vi "SerialSendHLcmd.vi"(0 "ASI stage":T1, 1 "Axis configuration":u16(ring) items=["No axis", "X", "Y", "Z", "XY", "XYZ"], 5 "Command":string, 7 "data in":cluster{"X in":dbl, "Y in":dbl, "Z in":dbl} {"Z in" format="%#.4f"; "Y in" format="%#.4f"; "X in" format="%#.4f"}, 11 "error in (no error)":errorcluster, 12 "Command type":enum16{"Query", "Where", "Imperative", "DU Y"}(ring)) -> (4 "Raw receive buffer":string, 6 "data out":cluster{"X out":dbl, "Y out":dbl, "Z out":dbl} {"Z out" format="%#.4f"; "Y out" format="%#.4f"; "X out" format="%#.4f"}, 15 "error out":errorcluster)   [LabVIEW 2010]
uses:
  stage properties.ctl
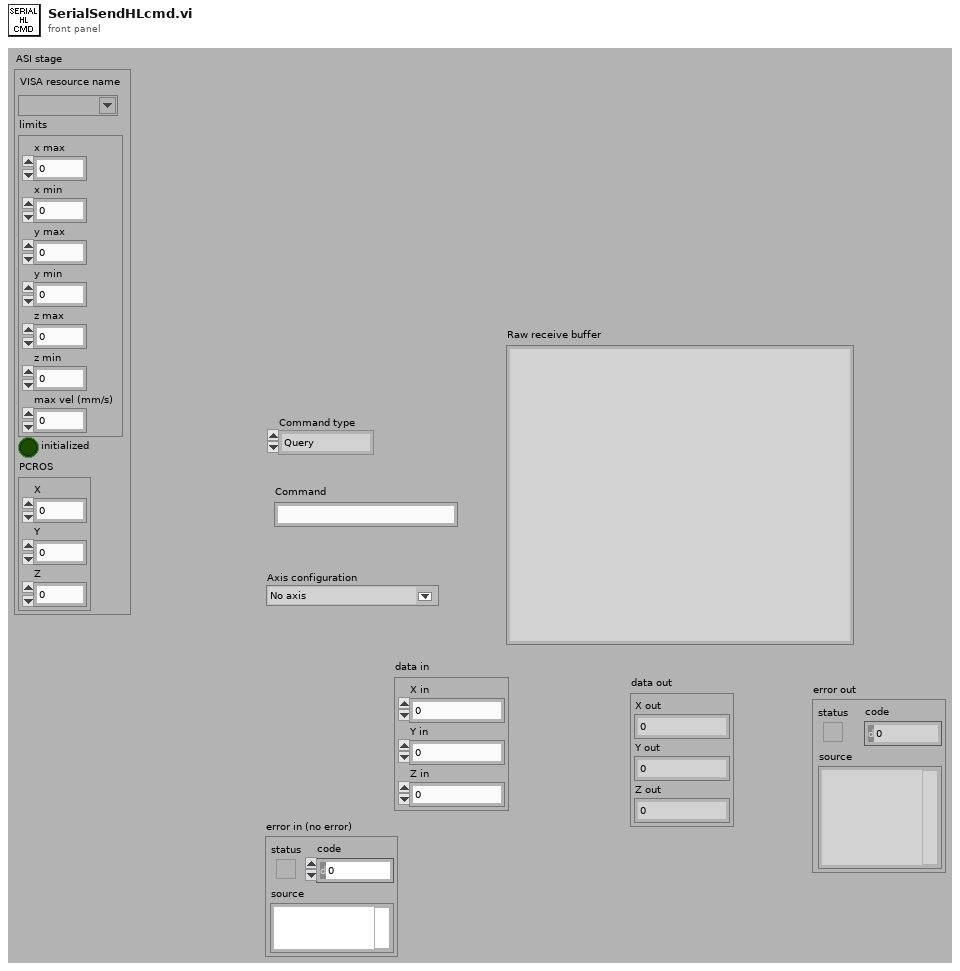
[diagram p1: front panel]
types:
  T1 = typedef "stage properties.ctl" = cluster{"VISA resource name":refnum<visa-resource-name>, "limits":cluster{"x max":dbl, "x min":dbl, "y max":dbl, "y min":dbl, "z max":dbl, "z min":dbl, "max vel (mm/s)":dbl}, "initialized":bool, "PCROS":cluster{"X":dbl, "Y":dbl, "Z":dbl}}
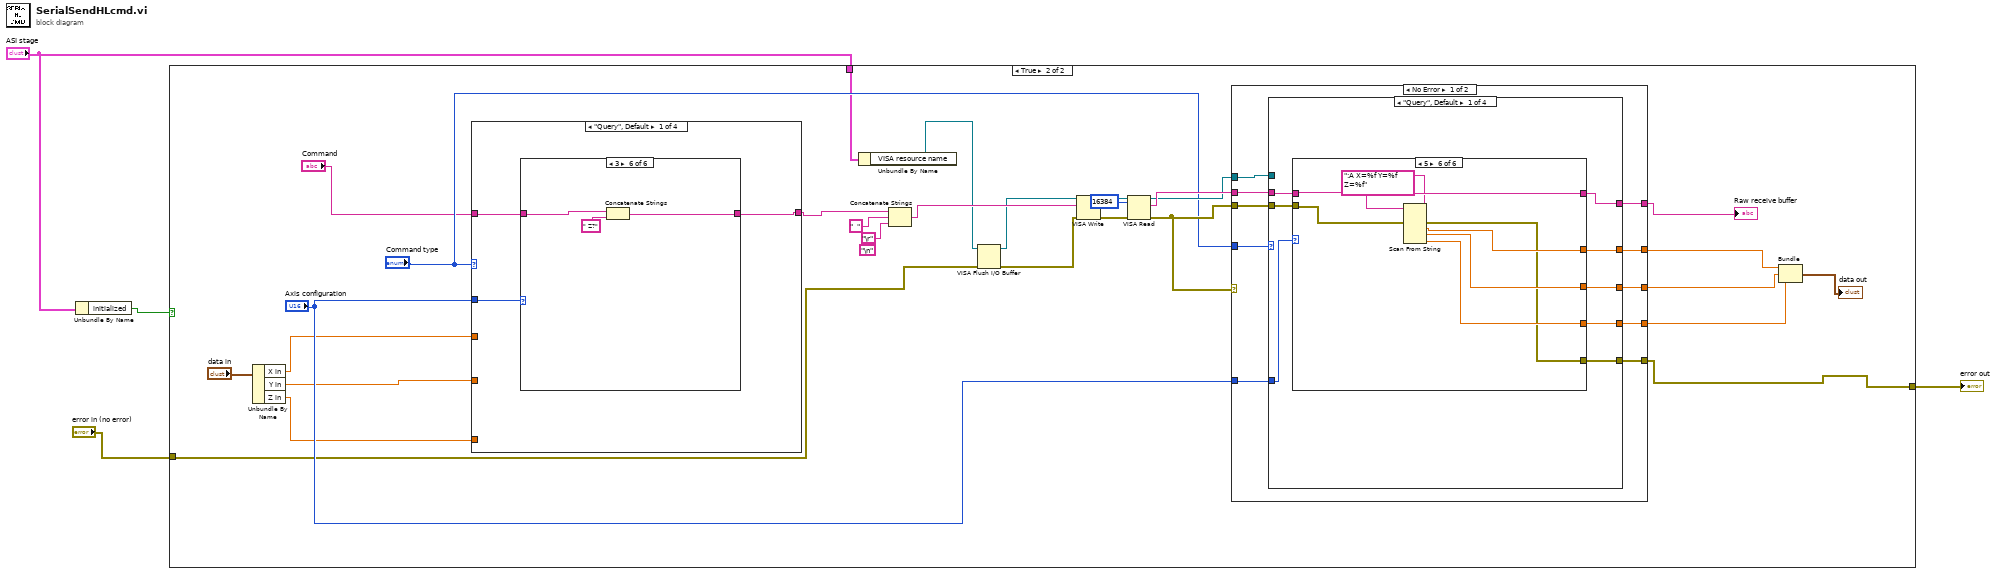
[diagram p0: block diagram]
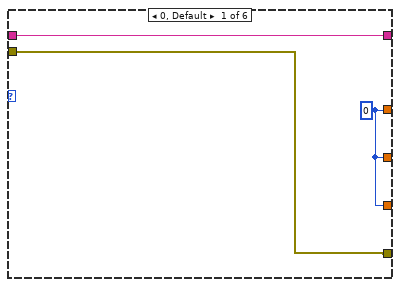
[diagram p3: hidden frame]
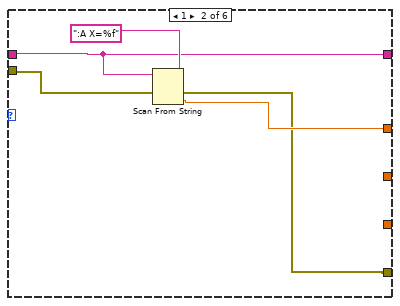
[diagram p4: hidden frame]
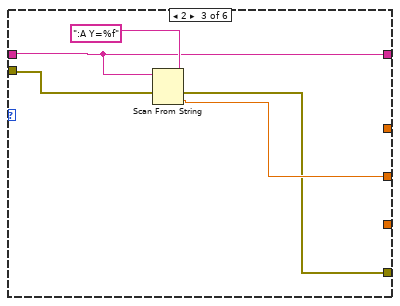
[diagram p5: hidden frame]
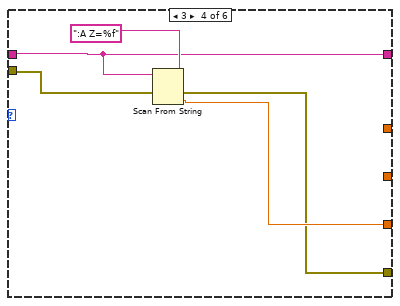
[diagram p6: hidden frame]
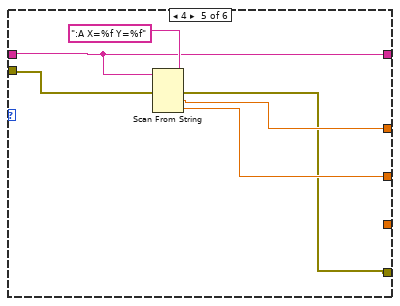
[diagram p7: hidden frame]
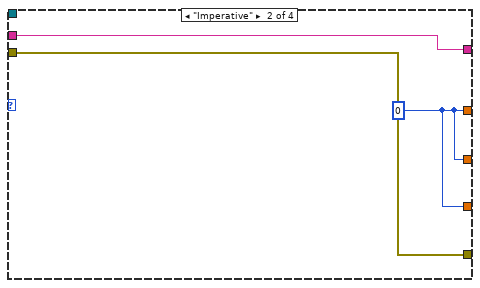
[diagram p8: hidden frame]
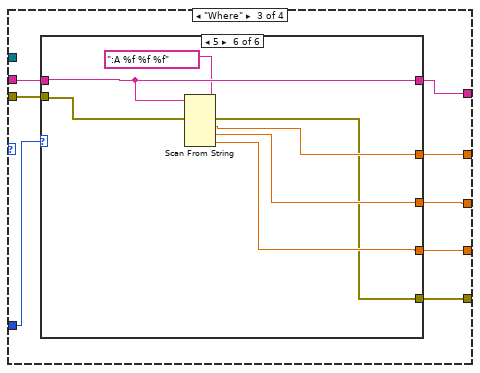
[diagram p9: hidden frame]
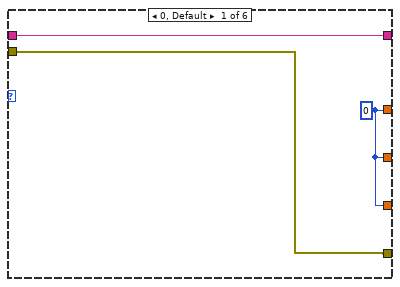
[diagram p10: hidden frame]
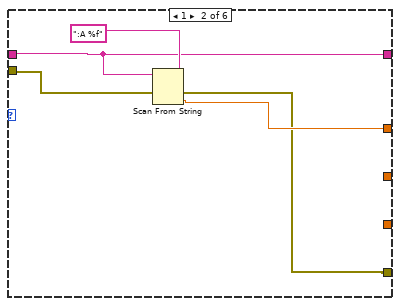
[diagram p11: hidden frame]
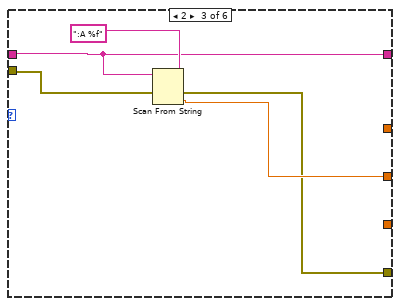
[diagram p12: hidden frame]
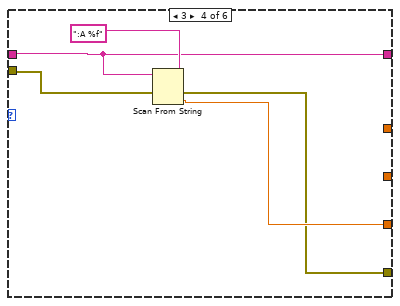
[diagram p13: hidden frame]
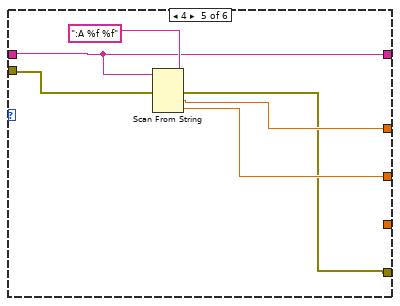
[diagram p14: hidden frame]
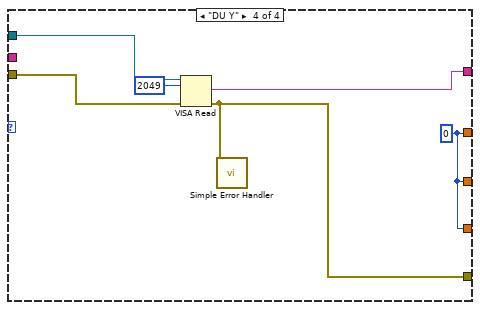
[diagram p15: hidden frame]
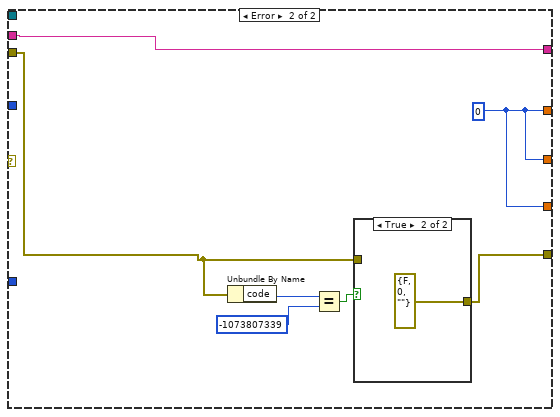
[diagram p16: hidden frame]
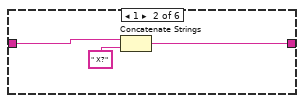
[diagram p19: hidden frame]
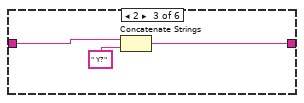
[diagram p20: hidden frame]
diagram:
  n1 = Unbundle By Name("ASI stage") -> ("initialized"=w1:bool)
  n2 = case shown="True" w1 {
    tunnel: "ASI stage" -> [_ w17]
    tunnel: [w5 w7] -> w4
    tunnel: "error in (no error)" -> [w5 w6]
    frame False {
    }
    frame True {
      (unwired) "\n"
      n3 = Unbundle By Name("data in") -> ("X in"=w15:dbl, "Y in"=w14:dbl, "Z in"=w13:dbl)
      n4 = case shown="\"Query\", Default" "Command type" {
        tunnel: "Command" -> [w141 w160 w183 _]
        tunnel: "Axis configuration" -> [w142 w161 w178 _]
        tunnel: w15 -> [_ _ w182 _]
        tunnel: w14 -> [_ _ w181 _]
        tunnel: w13 -> [_ _ w180 _]
        tunnel: [w140 w159 w179 "DU Y "] -> w33
        frame "Query", Default {
          n5 = case shown="3" w142 {
            tunnel: w141 -> [w143 w146 w149 w152 w155 w158]
            tunnel: [w143 w144 w147 w150 w153 w156] -> w140
            frame 0, Default {
            }
            frame 1 {
              n6 = Concatenate Strings "Concatenate Strings"(w146, " X?") -> (w144:string)
            }
            frame 2 {
              n7 = Concatenate Strings "Concatenate Strings"(w149, " Y?") -> (w147:string)
            }
            frame 4 {
              n8 = Concatenate Strings "Concatenate Strings"(w152, " X? Y?") -> (w150:string)
            }
            frame 5 {
              n9 = Concatenate Strings "Concatenate Strings"(w155, " X? Y? Z?") -> (w153:string)
            }
            frame 3 {
              n10 = Concatenate Strings "Concatenate Strings"(w158, " Z?") -> (w156:string)
            }
          }
        }
        frame "Where" {
          n11 = case shown="5" w161 {
            tunnel: w160 -> [w162 w165 w168 w171 w174 w177]
            tunnel: [w162 w163 w166 w169 w172 w175] -> w159
            frame 0, Default {
            }
            frame 1 {
              n12 = Concatenate Strings "Concatenate Strings"(w165, " X ") -> (w163:string)
            }
            frame 2 {
              n13 = Concatenate Strings "Concatenate Strings"(w168, " Y ") -> (w166:string)
            }
            frame 4 {
              n14 = Concatenate Strings "Concatenate Strings"(w171, " X Y") -> (w169:string)
            }
            frame 5 {
              n15 = Concatenate Strings "Concatenate Strings"(w174, " X Y Z ") -> (w172:string)
            }
            frame 3 {
              n16 = Concatenate Strings "Concatenate Strings"(w177, " Z") -> (w175:string)
            }
          }
        }
        frame "Imperative" {
          n17 = case shown="4" w178 {
            tunnel: w183 -> [w184 w188 w192 w196 w201 w207]
            tunnel: w182 -> [_ w186 _ _ w198 w204]
            tunnel: w181 -> [_ _ w189 _ w197 w203]
            tunnel: w180 -> [_ _ _ w193 _ w202]
            tunnel: [w184 w185 w190 w194 w199 w205] -> w179
            frame 0, Default {
            }
            frame 1 {
              n18 = Format Into String "Format Into String"(format string="  X=%7.4f", initial string=w188, w186) -> (resulting string=w185:string)  [unwired: 1 in, 1 out]
            }
            frame 2 {
              n19 = Format Into String "Format Into String"(format string="  Y=%7.4f", initial string=w192, w189) -> (resulting string=w190:string)  [unwired: 1 in, 1 out]
            }
            frame 3 {
              n20 = Format Into String "Format Into String"(format string=" Z=%7.4f", initial string=w196, w193) -> (resulting string=w194:string)  [unwired: 1 in, 1 out]
            }
            frame 4 {
              n21 = Format Into String "Format Into String"(format string=" X=%7.4f  Y=%7.4f", initial string=w201, w198, w197) -> (resulting string=w199:string)  [unwired: 1 in, 1 out]
            }
            frame 5 {
              n22 = Format Into String "Format Into String"(format string=" X=%7.4f  Y=%7.4f Z=%7.4f", initial string=w207, w204, w203, w202) -> (resulting string=w205:string)  [unwired: 1 in, 1 out]
            }
          }
        }
        frame "DU Y" {
        }
      }
      n23 = Unbundle By Name(w17) -> ("VISA resource name"=w8:refnum<visa-resource-name>)
      n24 = Concatenate Strings "Concatenate Strings"(w33, "  ", "\r") -> (w30:string)
      n25 = VISA Flush I/O Buffer(VISA resource name=w8, error in (no error)=w6) -> (VISA resource name out=w19:refnum<visa-resource-name>, error out=w29:errorcluster)  [unwired: 1 out]
      n26 = VISA Write(VISA resource name=w19, write buffer=w30, error in (no error)=w29) -> (VISA resource name out=w28:refnum<visa-resource-name>, error out=w27:errorcluster)  [unwired: 1 out]
      n27 = VISA Read(VISA resource name=w28, byte count=u32 16384, error in (no error)=w27) -> (VISA resource name out=w21:refnum<visa-resource-name>, read buffer=w26:string, error out=w22:errorcluster)  [unwired: 1 out]
      n28 = case shown="No Error" w22 {
        tunnel: w26 -> [w43 w136]
        tunnel: "Command type" -> [w42 _]
        tunnel: "Axis configuration" -> [w41 _]
        tunnel: [w40 w136] -> w24
        tunnel: [w39 w137] -> w12
        tunnel: [w38 w137] -> w11
        tunnel: [w37 w137] -> w10
        tunnel: w22 -> [w36 w131]
        tunnel: [w35 w133] -> w7
        tunnel: w21 -> [w34 _]
        frame No Error {
          n29 = case shown="\"Query\", Default" w42 {
            tunnel: w43 -> [w50 w85 w92 _]
            tunnel: w41 -> [w51 _ w93 _]
            tunnel: [w49 w85 w91 w128] -> w40
            tunnel: [w47 w84 w89 w127] -> w39
            tunnel: [w46 w84 w88 w127] -> w38
            tunnel: [w45 w84 w87 w127] -> w37
            tunnel: w36 -> [w48 w83 w90 w129]
            tunnel: [w44 w83 w86 w125] -> w35
            tunnel: w34 -> [_ _ _ w130]
            frame "Query", Default {
              n30 = case shown="5" w51 {
                tunnel: w50 -> [w54 w58 w63 w68 w74 w82]
                tunnel: [w54 w58 w63 w68 w74 w82] -> w49
                tunnel: w48 -> [w52 w57 w62 w67 w73 w81]
                tunnel: [w53 w56 _ _ w72 w80] -> w47
                tunnel: [w53 _ w61 _ w71 w79] -> w46
                tunnel: [w53 _ _ w66 _ w77] -> w45
                tunnel: [w52 w55 w60 w65 w70 w76] -> w44
                frame 0, Default {
                  w53 = 0
                }
                frame 1 {
                  n31 = Scan From String "Scan From String"(format string=":A X=%f", input string=w58, error in=w57) -> (error out=w55:errorcluster, output 1=w56:dbl)  [unwired: 2 in, 2 out]
                }
                frame 2 {
                  n32 = Scan From String "Scan From String"(format string=":A Y=%f", input string=w63, error in=w62) -> (error out=w60:errorcluster, output 1=w61:dbl)  [unwired: 2 in, 2 out]
                }
                frame 3 {
                  n33 = Scan From String "Scan From String"(format string=":A Z=%f", input string=w68, error in=w67) -> (error out=w65:errorcluster, output 1=w66:dbl)  [unwired: 2 in, 2 out]
                }
                frame 4 {
                  n34 = Scan From String "Scan From String"(format string=":A X=%f Y=%f", input string=w74, error in=w73) -> (error out=w70:errorcluster, output 1=w72:dbl, output 2=w71:dbl)  [unwired: 3 in, 2 out]
                }
                frame 5 {
                  n35 = Scan From String "Scan From String"(format string=":A X=%f Y=%f Z=%f", input string=w82, error in=w81) -> (error out=w76:errorcluster, output 1=w80:dbl, output 2=w79:dbl, output 3=w77:dbl)  [unwired: 4 in, 2 out]
                }
              }
            }
            frame "Imperative" {
              w84 = 0
            }
            frame "Where" {
              n36 = case shown="5" w93 {
                tunnel: w92 -> [w96 w100 w105 w110 w116 w124]
                tunnel: [w96 w100 w105 w110 w116 w124] -> w91
                tunnel: w90 -> [w94 w99 w104 w109 w115 w123]
                tunnel: [w95 w98 _ _ w114 w122] -> w89
                tunnel: [w95 _ w103 _ w113 w121] -> w88
                tunnel: [w95 _ _ w108 _ w119] -> w87
                tunnel: [w94 w97 w102 w107 w112 w118] -> w86
                frame 0, Default {
                  w95 = 0
                }
                frame 1 {
                  n37 = Scan From String "Scan From String"(format string=":A %f", input string=w100, error in=w99) -> (error out=w97:errorcluster, output 1=w98:dbl)  [unwired: 2 in, 2 out]
                }
                frame 2 {
                  n38 = Scan From String "Scan From String"(format string=":A %f", input string=w105, error in=w104) -> (error out=w102:errorcluster, output 1=w103:dbl)  [unwired: 2 in, 2 out]
                }
                frame 3 {
                  n39 = Scan From String "Scan From String"(format string=":A %f", input string=w110, error in=w109) -> (error out=w107:errorcluster, output 1=w108:dbl)  [unwired: 2 in, 2 out]
                }
                frame 4 {
                  n40 = Scan From String "Scan From String"(format string=":A %f %f", input string=w116, error in=w115) -> (error out=w112:errorcluster, output 1=w114:dbl, output 2=w113:dbl)  [unwired: 3 in, 2 out]
                }
                frame 5 {
                  n41 = Scan From String "Scan From String"(format string=":A %f %f %f", input string=w124, error in=w123) -> (error out=w118:errorcluster, output 1=w122:dbl, output 2=w121:dbl, output 3=w119:dbl)  [unwired: 4 in, 2 out]
                }
              }
            }
            frame "DU Y" {
              w127 = 0
              n42 = VISA Read(VISA resource name=w130, byte count=u32 2049, error in (no error)=w129) -> (read buffer=w128:string, error out=w125:errorcluster)  [unwired: 2 out]
              n43 = call <vilib>:"Simple Error Handler.vi"("error in (no error)"=w125) -> ()  [unwired: 1 in, 8 out]
            }
          }
        }
        frame Error {
          w137 = 0
          n44 = Unbundle By Name(w131) -> ("code"=w135:i32)
          n45 = Equal?(x=w135, y=-1073807339) -> (x = y?=w132:bool)
          n46 = case shown="True" w132 {
            tunnel: [w138 errorcluster {"status"=FALSE, "code"=0, "source"=""}] -> w133
            tunnel: w131 -> [w138 _]
            frame False {
            }
            frame True {
            }
          }
        }
      }
      "Raw receive buffer" <- w24
      n47 = Bundle(w12, w11, w10) -> (→"data out":cluster{dbl, dbl, dbl})  [unwired: 1 in]
    }
  }
  "error out" <- w4
